vi "DMMP_GetComments.vi"(3 "Input DMMP":refnum<class "DMMP.lvclass">) -> (0 "Comments":string, 1 "Output DMMP":refnum<class "DMMP.lvclass">)   [LabVIEW 2014, in "DMMP.lvclass"]
uses:
  DMMP.lvclass
  DMMP.lvclass/DMMP.ctl
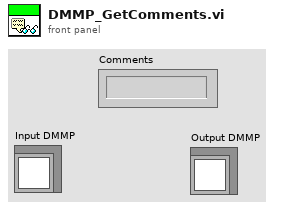
[diagram p1: front panel]
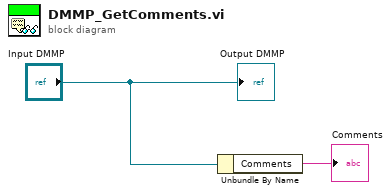
[diagram p0: block diagram]
diagram:
  n1 = Unbundle By Name("Input DMMP") -> ("Comments"=→"Comments":string)
  "Output DMMP" <- "Input DMMP"
